vi "MCP Current Position.vi"(3 "error in (no error)":errorcluster, 4 "Initial Couter Reading":dbl=-1125000.0 format="%.2f", 5 "Initial Stepper Position":i32=-1125000) -> (0 "error out":errorcluster, 1 "Current Couter Reading":dbl=-1125000.0 format="%.2f", 2 "Current Stepper Position":i32=-1125000)   [LabVIEW 2019]
uses:
  Globals and TypeDefs/Global Varibal Control.vi
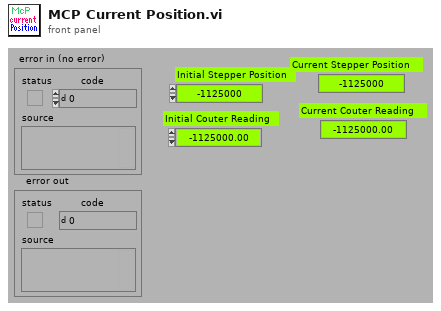
[diagram p1: front panel]
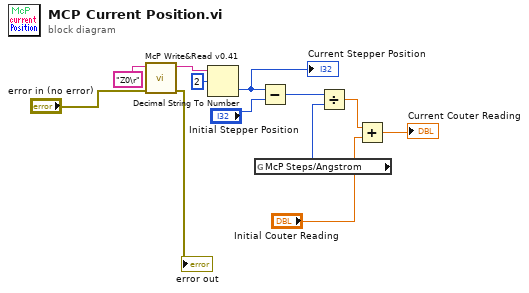
[diagram p0: block diagram]
diagram:
  n1 = call "McP Write&Read v0.41.vi"("error in (no error)"="error in (no error)", "Write String"="Z0\r") -> ("error out"=→"error out":errorcluster, "Read String\nshows:"=w11:string)  [unwired: 2 in, 3 out]
  n2 = Decimal String To Number(string=w11, offset=2) -> (number=w1:i32)  [unwired: 1 in, 1 out]
  "Current Stepper Position" <- w1
  n3 = global read "Global Varibal Control.vi" "McP Steps/Angstrom"() -> (w7:i32)
  n4 = Subtract(x=w1, y="Initial Stepper Position") -> (x-y=w9:i32)
  n5 = Divide(x=w9, y=w7) -> (x/y=w8:dbl)
  n6 = Add(x=w8, y="Initial Couter Reading") -> (x+y=→"Current Couter Reading":dbl)
